vi "校准设置页.vi"() -> ()   [LabVIEW 2016, in "斯坦道氨氮V2.lvlib"]
uses:
  <vilib>/ptbypt/NI_PtbyPt.lvlib
panel:
  in  "校准任务":bool
  in  "历史数据导入":T1(radio)
  out "刷新时间":string
  out "模型刷新":bool
  in  "校准按钮":T1(radio)
  in  "仪器写入":bool
  in  "辅助计算":bool
  in  "曲线模型":T2={"标液浓度1"=0.0, "测量吸光度1"=0.0, "样品1启用"=FALSE, "标液浓度2"=0.0, "测量吸光度2"=0.0, "样品2启用"=FALSE, "标液浓度3"=0.0, "测量吸光度3"=0.0, "样品3启用"=FALSE, "标液浓度4"=0.0, "测量吸光度4"=0.0, "样品4启用"=FALSE, "标液浓度5"=0.0, "测量吸光度5"=0.0, "样品5启用"=FALSE, "模型"=enum."线性", "精度"=4.0, "XY图"=[], "拟合公式"="", "r^2"=0.0, "标样一校准时间"=timestamp(0 s since 1904-01-01), "标样二校准时间"=timestamp(0 s since 1904-01-01), "标样三校准时间"=timestamp(0 s since 1904-01-01), "标样四校准时间"=timestamp(0 s since 1904-01-01), "标样五校准时间"=timestamp(0 s since 1904-01-01), "二次方程"={"c"=0.0, "x"=0.0, "x^2"=0.0}, "标定时间"=timestamp(0 s since 1904-01-01)} {"标定时间" format="%<%y/%m/%d %H:%M:%S>T"; "标样五校准时间" format="%<%y/%m/%d %H:%M:%S>T"; "标样四校准时间" format="%<%y/%m/%d %H:%M:%S>T"; "标样三校准时间" format="%<%y/%m/%d %H:%M:%S>T"; "标样二校准时间" format="%<%y/%m/%d %H:%M:%S>T"; "标样一校准时间" format="%<%y/%m/%d %H:%M:%S>T"; "r^2" format="%.7f"; "测量吸光度5" format="%#.6f"; "测量吸光度4" format="%#.6f"; "测量吸光度3" format="%#.6f"; "测量吸光度2" format="%#.6f"; "测量吸光度1" format="%#.6f"}
  in  "测量模式":enum16{"跨度核查", "水样测量", "零点核查", "标样核查", "加标回收"}(ring)
  in  "参数下拉列表":u16(ring) items=["氨氮"=3, "CODMn"=21]
  in  "量程下拉列表":enum16{"低量程", "高量程"}(ring)
  # "校准时间"
  # "标液浓度"
  # "吸光值"
  # "标样一"
  # "标样二"
  # "标样三"
  # "零点"
  # "跨度"
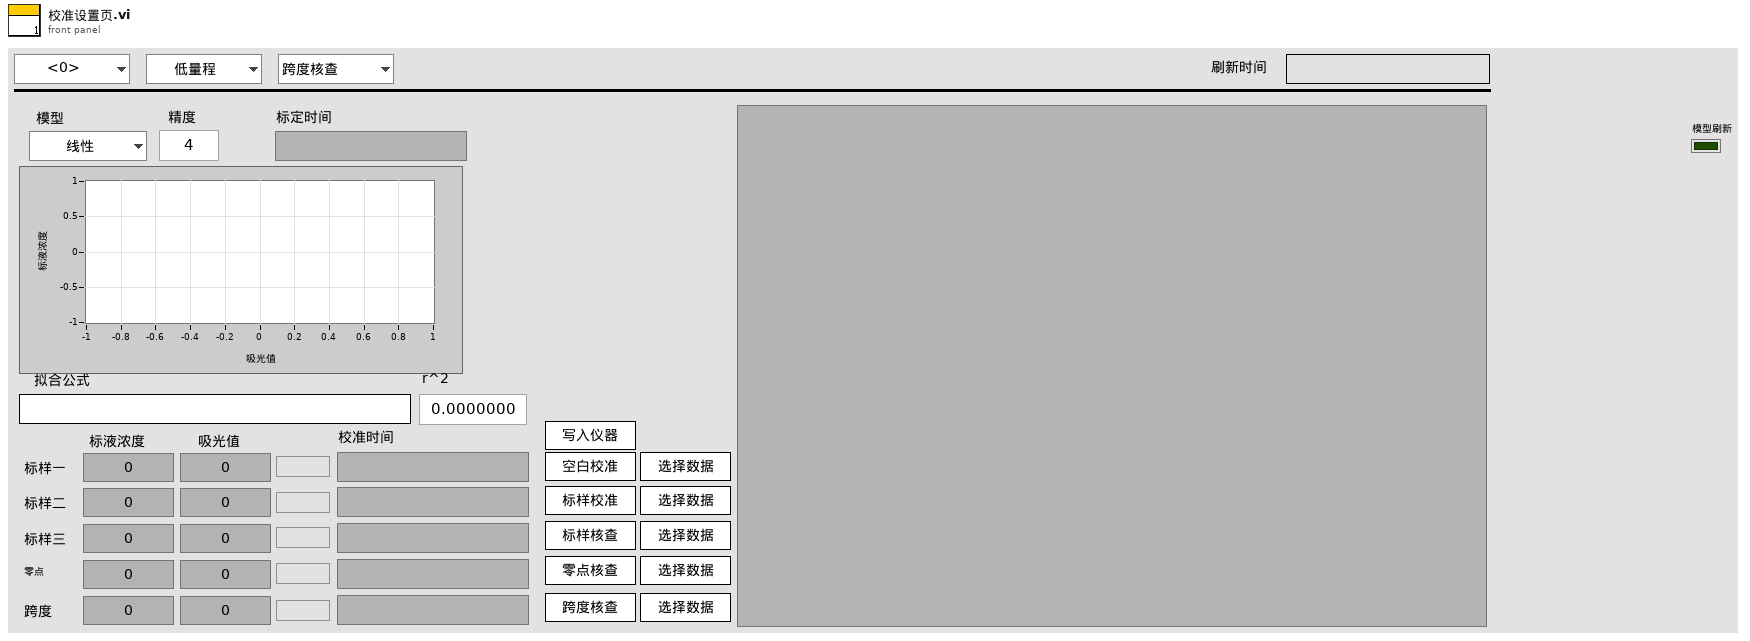
[diagram p1: front panel]
types:
  T1 = enum32{"未选择", "空白校准", "标样校准", "标样核查", "零点核查", "跨度核查"}
  T2 = cluster{"标液浓度1":dbl, "测量吸光度1":dbl, "样品1启用":bool, "标液浓度2":dbl, "测量吸光度2":dbl, "样品2启用":bool, "标液浓度3":dbl, "测量吸光度3":dbl, "样品3启用":bool, "标液浓度4":dbl, "测量吸光度4":dbl, "样品4启用":bool, "标液浓度5":dbl, "测量吸光度5":dbl, "样品5启用":bool, "模型":enum32{"线性", "多项式"}, "精度":dbl, "XY图":cluster{"X Values":dbl[], "Y Values":dbl[]}[], "拟合公式":string, "r^2":dbl, "标样一校准时间":timestamp, "标样二校准时间":timestamp, "标样三校准时间":timestamp, "标样四校准时间":timestamp, "标样五校准时间":timestamp, "二次方程":cluster{"c":dbl, "x":dbl, "x^2":dbl}, "标定时间":timestamp}
  T3 = typedef "斯坦道氨氮V2.lvlib/校准任务.ctl" = cluster{"id":u16, "任务类型":enum16{"未选择", "空白校准", "标样校准", "标样核查", "零点核查", "跨度核查"}, "量程下拉列表":enum16{"低量程", "高量程"}, "状态":enum16{"已执行", "待执行", "执行中", "停止"}, "标液浓度":dbl, "吸光值":dbl, "校准时间":timestamp}
  T4 = enum8{"Enabled", "Disabled", "Disabled and Grayed Out"}
  T5 = enum16{"跨度核查", "水样测量", "零点核查", "标样核查", "加标回收", "快捷测试", "空白校准", "标样校准"}
  T6 = typedef "LVStringsAndValuesArrayTypeDef_U16.ctl" = cluster{"String":string, "Value":u16}[]
  T7 = cluster{"标液浓度1":dbl, "测量吸光度1":dbl, "样品1启用":bool, "标液浓度2":dbl, "测量吸光度2":dbl, "样品2启用":bool, "标液浓度3":dbl, "测量吸光度3":dbl, "样品3启用":bool, "标液浓度4":dbl, "测量吸光度4":dbl, "样品4启用":bool, "标液浓度5":dbl, "测量吸光度5":dbl, "样品5启用":bool, "模型":enum32{"线性", "多项式"}, "精度":dbl, "XY图":cluster{"X Values":dbl[], "Y Values":dbl[]}[], "拟合公式":string, "r^2":dbl, "标样一校准时间":timestamp, "标样二校准时间":timestamp, "标样三校准时间":timestamp, "标样四校准时间":timestamp, "标样五校准时间":timestamp, "二次方程":cluster{"c":dbl, "x":dbl, "x^2":dbl}, "标定时间":timestamp}[]
  T8 = cluster{"时间":timestamp, "标液值":dbl, "检测值":dbl, "吸光值":dbl}
  T9 = enum32{"Bad", "Idle", "Run top level", "Running"}
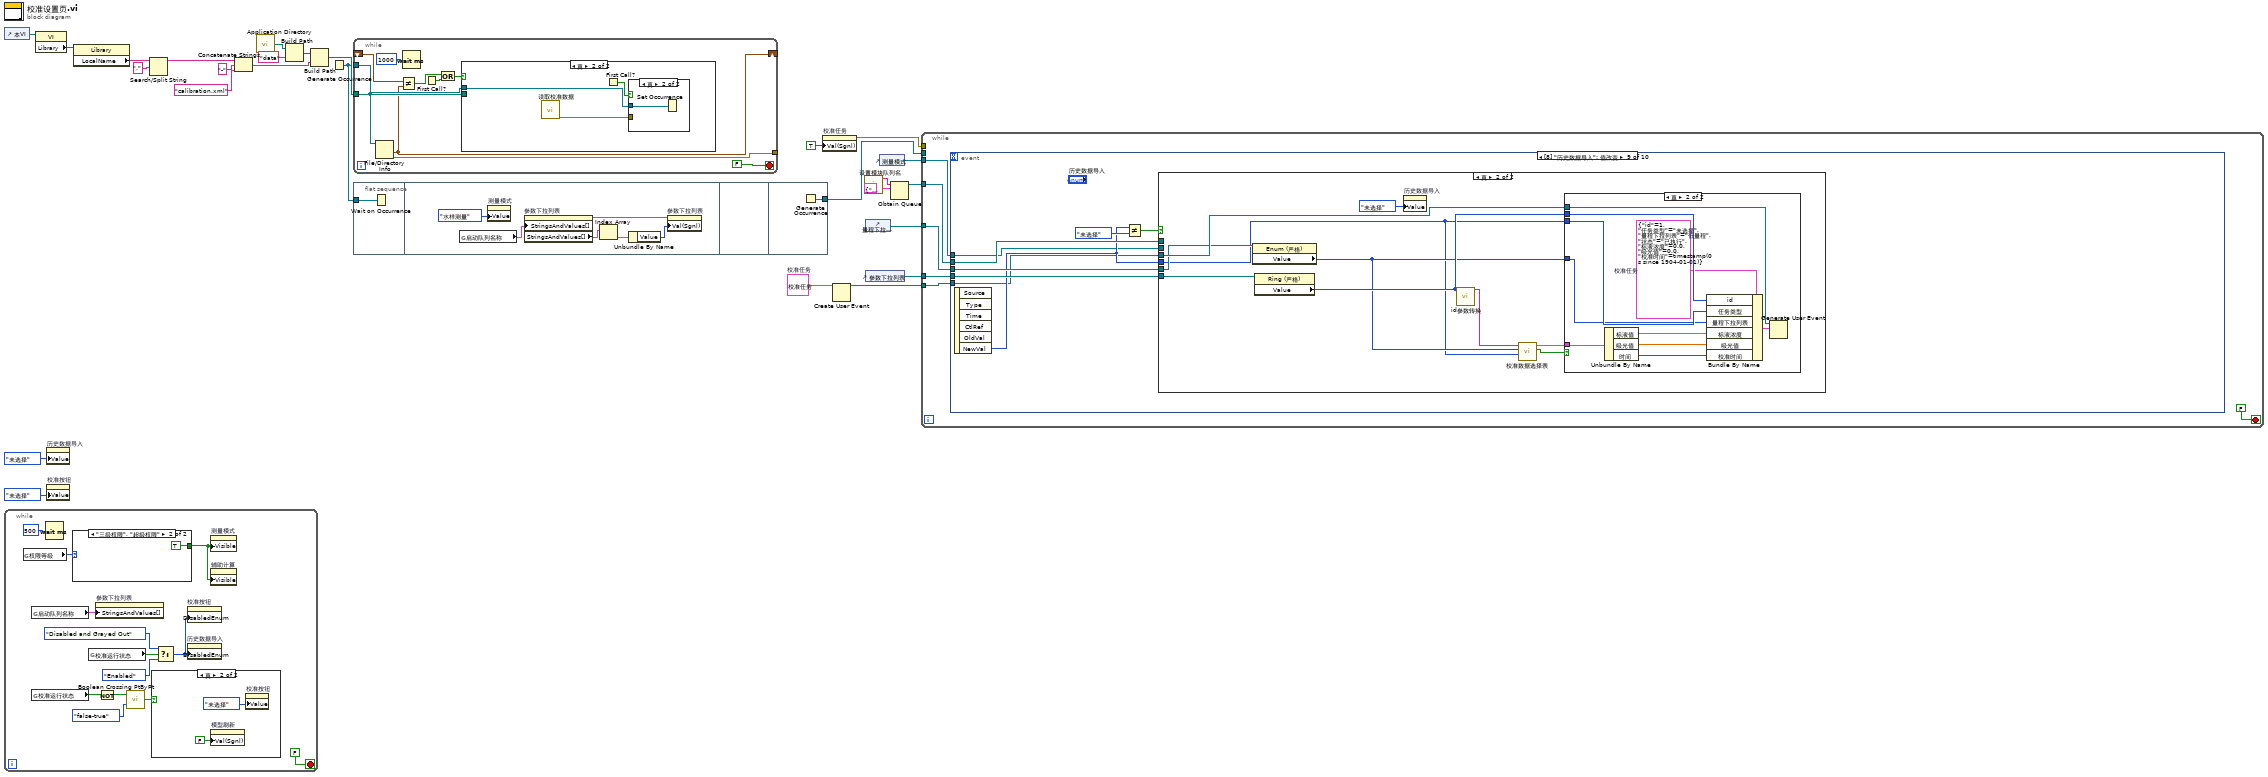
[diagram p0: block diagram]
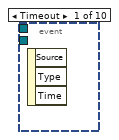
[diagram p4: hidden frame]
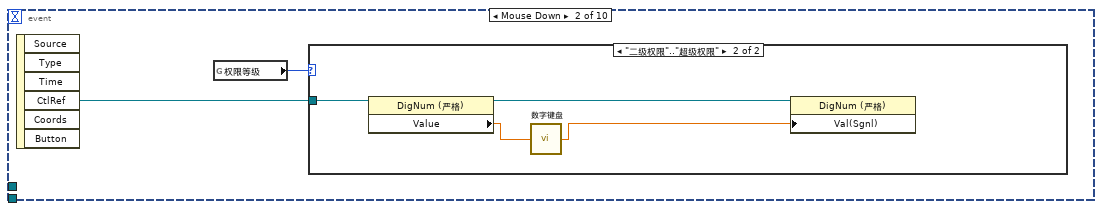
[diagram p5: hidden frame]
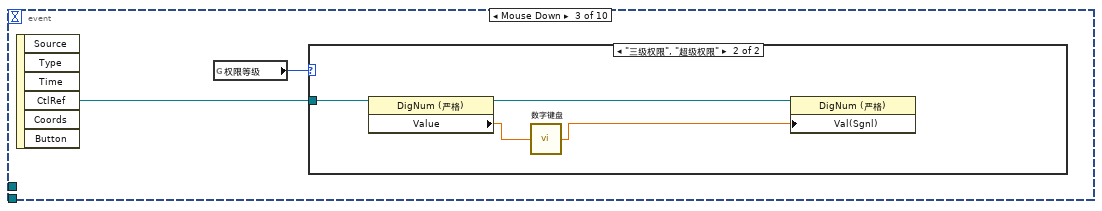
[diagram p7: hidden frame]
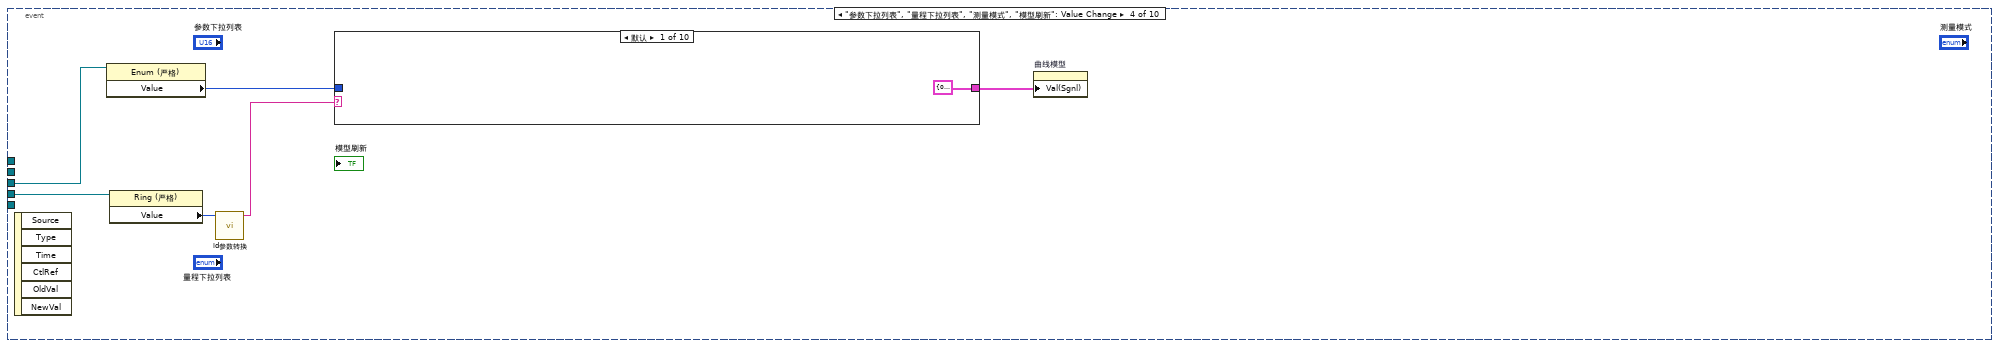
[diagram p9: hidden frame]
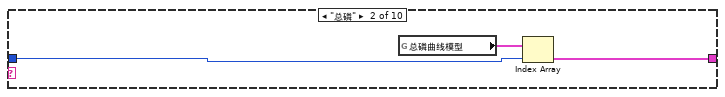
[diagram p10: hidden frame]
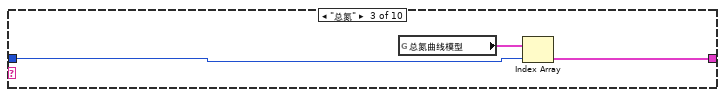
[diagram p11: hidden frame]
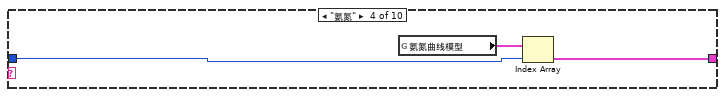
[diagram p12: hidden frame]
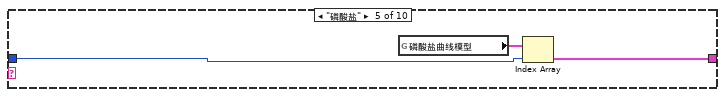
[diagram p13: hidden frame]
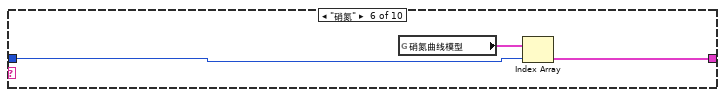
[diagram p14: hidden frame]
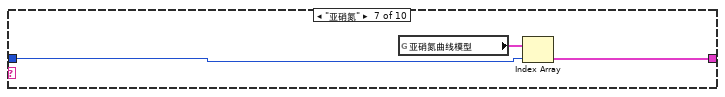
[diagram p15: hidden frame]
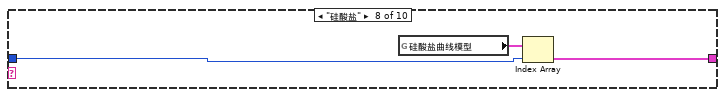
[diagram p16: hidden frame]
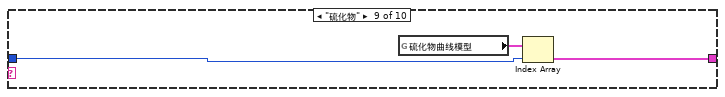
[diagram p17: hidden frame]
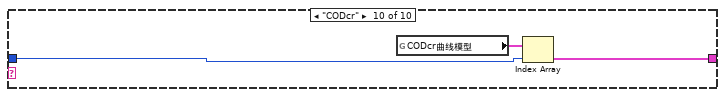
[diagram p18: hidden frame]
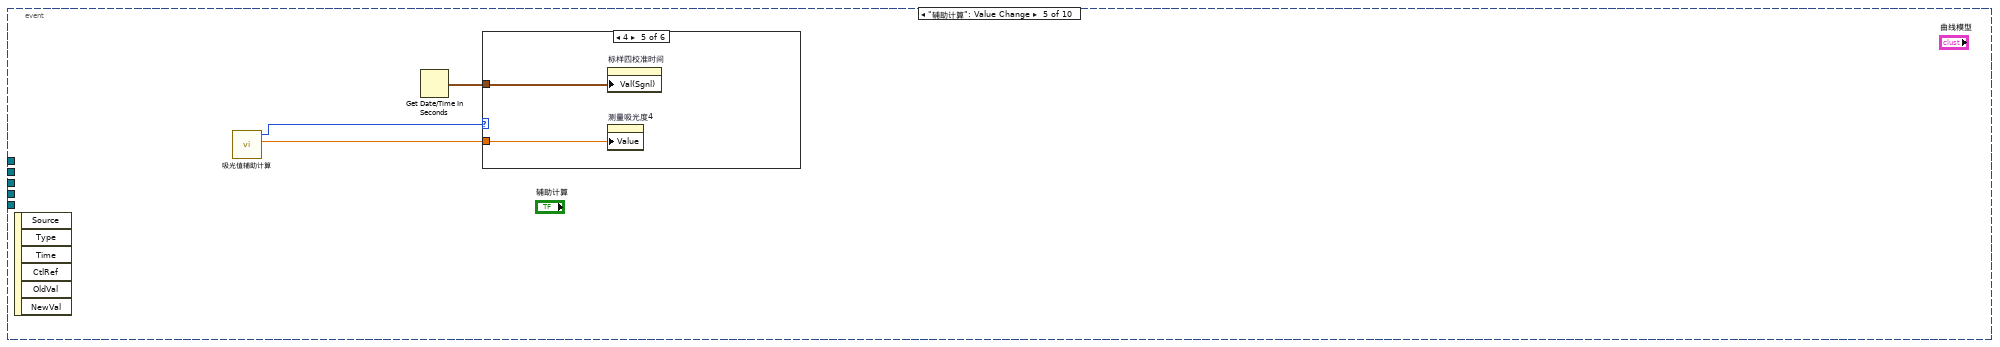
[diagram p19: hidden frame]
diagram:
  w3 = T3 {"id"=1, "任务类型"=enum."未选择", "量程下拉列表"=enum."低量程", "状态"=enum."已执行", "标液浓度"=0.0, "吸光值"=0.0, "校准时间"=timestamp(0 s since 1904-01-01)}  # 校准任务
  n1 = control-ref of="本VI"() -> (w14:refnum<vi>)
  n2 = while {
    stop <- FALSE stop-if-true
    n3 = global read "VAR总磷总氮全局变量.vi" "权限等级"() -> (w37:enum16{"一级权限", "二级权限", "三级权限", "超级权限"})
    n4 = global read "总磷总氮断电保存全局变量.vi" "启动队列名称"() -> (w34:cluster{"String":string, "Value":u16}[])
    n5 = global read "VAR总磷总氮全局变量.vi" "校准运行状态"() -> (w33:bool)
    n6 = Wait (ms)(milliseconds to wait=u32 500 ("等待时间（毫秒）")) -> ()  [unwired: 1 out]
    n7 = case shown="\"三级权限\", \"超级权限\"" w37 {
      tunnel: [_ TRUE ("可见")] -> w27
      frame "一级权限", Default {
        n8 = property on="测量模式" class="Enum (严格)"("Value"=T5."水样测量" ("测量模式")) -> ()  [unwired: 2 in, 2 out]
      }
      frame "三级权限", "超级权限" {
      }
    }
    n9 = global read "VAR总磷总氮全局变量.vi" "校准运行状态"() -> (w31:bool)
    n10 = property on="参数下拉列表" class="Ring (严格)"("StringsAndValues[]"=w34) -> ()  [unwired: 2 in, 2 out]
    n11 = Not(x=w33) -> (.not. x?=w32:bool)
    n12 = call <vilib>:"Boolean Crossing PtByPt.vi"("direction"=enum16{"either", "false-true", "true-false"}."false-true", "input"=w32) -> ("crossing"=w35:bool)  [unwired: 1 in]
    n13 = case shown="真" w35 {
      frame False {
      }
      frame True {
        n14 = property on="模型刷新" class="Bool (严格)"("Val(Sgnl)"=FALSE ("值(信号)")) -> ()  [unwired: 2 in, 2 out]
        n15 = property on="校准按钮" class="RadioBtnsControl (严格)"("Value"=T1."未选择" ("校准按钮")) -> ()  [unwired: 2 in, 2 out]
      }
    }
    n16 = Select(t=T4."Disabled and Grayed Out" ("禁用"), s=w31, f=T4."Enabled" ("禁用")) -> (s? t:f=w29:T4)
    n17 = property on="校准按钮" class="RadioBtnsControl (严格)"("DisabledEnum"=w29) -> ()  [unwired: 2 in, 2 out]
    n18 = property on="历史数据导入" class="RadioBtnsControl (严格)"("DisabledEnum"=w29) -> ()  [unwired: 2 in, 2 out]
    n19 = property on="测量模式" class="Enum (严格)"("Visible"=w27) -> ()  [unwired: 2 in, 2 out]
    n20 = property on="辅助计算" class="Bool"("Visible"=w27) -> ()  [unwired: 2 in, 2 out]
  }
  n21 = property class="VI"(reference=w14) -> ("Library"=w15:refnum<vi>)  [unwired: 1 in, 2 out]
  n22 = property on="历史数据导入" class="RadioBtnsControl (严格)"("Value"=T1."未选择" ("历史数据导入")) -> ()  [unwired: 2 in, 2 out]
  n23 = property on="校准按钮" class="RadioBtnsControl (严格)"("Value"=T1."未选择" ("校准按钮")) -> ()  [unwired: 2 in, 2 out]
  n24 = property class="Library"(reference=w15) -> ("LocalName"=w12:string)  [unwired: 1 in, 2 out]
  n25 = Search/Split String(string=w12, search string/char (-)="." ("搜索字符串/字符(-)")) -> (substring before match=w10:string)  [unwired: 1 in, 2 out]
  n26 = Concatenate Strings(w10, "-" ("字符串"), "calibration.xml" ("名称或相对路径")) -> (w7:string)
  n27 = call <vilib>:"Application Directory.vi"() -> ("Application Directory"=w16:path)
  n28 = Build Path(base path=w16, name or relative path="data" ("名称或相对路径")) -> (appended path=w13:path)
  n29 = Build Path(base path=w13, name or relative path=w7) -> (appended path=w6:path)
  n30 = Generate Occurrence() -> (w5:refnum<k4>)
  n31 = while {
    shift-right: [w44] -> _
    shift-left: _ -> [w52]
    tunnel: w6 -> [w50]
    tunnel: [w48] -> _
    tunnel: w5 -> [w47]
    stop <- FALSE stop-if-true
    n32 = File/Directory Info(path=w50) -> (last mod=w44:timestamp, error out=w48:errorcluster)  [unwired: 1 in, 5 out]
    n33 = Not Equal?(x=w52, y=w44) -> (x != y?=w51:bool)
    n34 = Wait (ms)(milliseconds to wait=u32 1000 ("等待时间（毫秒）")) -> ()  [unwired: 1 out]
    n35 = First Call?() -> (First Call?: T/F=w45:bool)
    n36 = Or(x=w51, y=w45) -> (x .or. y?=w46:bool)
    n37 = case shown="真" w46 {
      tunnel: w50 -> [_ _]
      tunnel: w47 -> [_ w56]
      frame False {
      }
      frame True {
        n38 = call "读取校准数据.vi"() -> ("错误输出"=w55:errorcluster)  [unwired: 11 in]
        n39 = First Call?() -> (First Call?: T/F=w54:bool)
        n40 = case shown="真" w54 {
          tunnel: w56 -> [_ w57]
          tunnel: w55 -> [_ _]
          frame False {
          }
          frame True {
            n41 = Set Occurrence(w57) -> ()
          }
        }
      }
    }
  }
  n42 = flat-sequence {
    tunnel: w5 -> [w58]
    tunnel: [w65] -> w26
    frame #0 {
      n43 = Wait on Occurrence(2:w58) -> ()  [unwired: 2 in, 1 out]
    }
    frame #1 {
      n44 = global read "总磷总氮断电保存全局变量.vi" "启动队列名称"() -> (w60:cluster{"String":string, "Value":u16}[])
      n45 = property on="测量模式" class="Enum (严格)"("Value"=T5."水样测量" ("测量模式")) -> ()  [unwired: 2 in, 2 out]
      n46 = property on="参数下拉列表" class="Ring (严格)"("StringsAndValues[]"=w60) -> (error out=w63:errorcluster, "StringsAndValues[]"=w61:T6)  [unwired: 2 in, 1 out]
      n47 = Index Array(array=w61) -> (element=w62:cluster{"String":string, "Value":u16})  [unwired: 1 in]
      n48 = Unbundle By Name(w62) -> ("Value"=w64:u16)
      n49 = property on="参数下拉列表" class="Ring (严格)"(error in=w63, "Val(Sgnl)"=w64) -> ()  [unwired: 1 in, 2 out]
    }
    frame #2 {
    }
    frame #3 {
      n50 = Generate Occurrence() -> (w65:refnum<k4>)
    }
  }
  n51 = property on="校准任务" class="Bool (严格)"("Val(Sgnl)"=TRUE ("值(信号)")) -> (error out=w2:errorcluster)  [unwired: 2 in, 1 out]
  n52 = Create User Event(user event datatype=w3) -> (user event=w4:refnum<user-event>)  [unwired: 1 in, 1 out]
  n53 = call "设置模块队列名.vi"() -> ("Msg"=w24:string)  [unwired: 5 in]
  n54 = control-ref of="量程下拉列表"() -> (w19:refnum<vi>)
  n55 = control-ref of="参数下拉列表"() -> (w21:refnum<vi>)
  n56 = control-ref of="测量模式"() -> (w20:refnum<vi>)
  n57 = Obtain Queue(name (unnamed)=w24, element data type=cluster{"命令":string, "data":variant} {"命令"="", "data"=variant}) -> (queue out=w23:refnum<queue>)  [unwired: 3 in, 2 out]
  n58 = while {
    tunnel: w26 -> [_]
    tunnel: w21 -> [w70]
    tunnel: w20 -> [w69]
    tunnel: w19 -> [w68]
    tunnel: w23 -> [w67]
    tunnel: w4 -> [w66]
    tunnel: w2 -> [_]
    stop <- FALSE stop-if-true
    n59 = event shown="[8] \"历史数据导入\": 值改变" {
      selector: _ -> [_ _ _ _ _ _ _ _ _ _]
      dyn-events: _ -> [_ _ _ _ _ _ _ _ _ _]
      timeout: _ -> [_ _ _ _ _ _ _ _ _ _]
      tunnel: w70 -> [_ _ _ w88 _ w143 w188 w242 w270 _]
      tunnel: w69 -> [_ _ _ _ _ w141 _ w237 w265 _]
      tunnel: w68 -> [_ _ _ w86 _ w139 w186 w241 w269 _]
      tunnel: w67 -> [_ _ _ _ _ _ _ w243 w271 _]
      tunnel: w66 -> [_ _ _ _ _ _ _ w236 w264 w293]
      event Timeout {
        n60 = event-data() -> ()  [unwired: 1 in, 3 out]
      }
      event "曲线模型.标液浓度1", "曲线模型.标液浓度2", "曲线模型.标液浓度3", "曲线模型.标液浓度4", "曲线模型.标液浓度5", "曲线模型.精度": Mouse Down {
        n61 = event-data() -> ("CtlRef"=w73:refnum<vi>)  [unwired: 1 in, 5 out]
        n62 = global read "VAR总磷总氮全局变量.vi" "权限等级"() -> (w72:enum16{"一级权限", "二级权限", "三级权限", "超级权限"})
        n63 = case shown="\"二级权限\"..\"超级权限\"" w72 {
          tunnel: w73 -> [_ w77]
          frame "一级权限", Default {
          }
          frame "二级权限".."超级权限" {
            n64 = property class="DigNum (严格)"(reference=w77) -> (reference out=w75:refnum<vi>, "Value"=w76:dbl)  [unwired: 1 in, 1 out]
            n65 = call "数字键盘.vi"("OldNumber"=w76) -> ("NewNumber"=w74:dbl)
            n66 = property class="DigNum (严格)"(reference=w75, "Val(Sgnl)"=w74) -> ()  [unwired: 1 in, 2 out]
          }
        }
      }
      event "曲线模型.测量吸光度1", "曲线模型.测量吸光度2", "曲线模型.测量吸光度3", "曲线模型.测量吸光度4", "曲线模型.测量吸光度5": Mouse Down {
        n67 = event-data() -> ("CtlRef"=w79:refnum<vi>)  [unwired: 1 in, 5 out]
        n68 = global read "VAR总磷总氮全局变量.vi" "权限等级"() -> (w78:enum16{"一级权限", "二级权限", "三级权限", "超级权限"})
        n69 = case shown="\"三级权限\", \"超级权限\"" w78 {
          tunnel: w79 -> [_ w83]
          frame "一级权限", Default {
          }
          frame "三级权限", "超级权限" {
            n70 = property class="DigNum (严格)"(reference=w83) -> (reference out=w81:refnum<vi>, "Value"=w82:dbl)  [unwired: 1 in, 1 out]
            n71 = call "数字键盘.vi"("OldNumber"=w82) -> ("NewNumber"=w80:dbl)
            n72 = property class="DigNum (严格)"(reference=w81, "Val(Sgnl)"=w80) -> ()  [unwired: 1 in, 2 out]
          }
        }
      }
      event "参数下拉列表", "量程下拉列表", "测量模式", "模型刷新": Value Change {
        n73 = event-data() -> ()  [unwired: 1 in, 6 out]
        n74 = property class="Enum (严格)"(reference=w86) -> ("Value"=w84:enum16{"低量程", "高量程"})  [unwired: 1 in, 2 out]
        n75 = property class="Ring (严格)"(reference=w88) -> ("Value"=w89:u16)  [unwired: 1 in, 2 out]
        n76 = call "id参数转换.vi"("id"=w89) -> ("table输出"=w87:string)  [unwired: 9 in, 1 out]
        n77 = case shown="默认" w87 {
          tunnel: w84 -> [_ w91 w94 w97 w100 w103 w106 w109 w112 w115]
          tunnel: [T2 {"标液浓度1"=0.0, "测量吸光度1"=0.0, "样品1启用"=FALSE, "标液浓度2"=0.0, "测量吸光度2"=0.0, "样品2启用"=FALSE, "标液浓度3"=0.0, "测量吸光度3"=0.0, "样品3启用"=FALSE, "标液浓度4"=0.0, "测量吸光度4"=0.0, "样品4启用"=FALSE, "标液浓度5"=0.0, "测量吸光度5"=0.0, "样品5启用"=FALSE, "模型"=enum."线性", "精度"=0.0, "XY图"=[], "拟合公式"="", "r^2"=0.0, "标样一校准时间"=timestamp(0 s since 1904-01-01), "标样二校准时间"=timestamp(0 s since 1904-01-01), "标样三校准时间"=timestamp(0 s since 1904-01-01), "标样四校准时间"=timestamp(0 s since 1904-01-01), "标样五校准时间"=timestamp(0 s since 1904-01-01), "二次方程"={"c"=0.0, "x"=0.0, "x^2"=0.0}, "标定时间"=timestamp(0 s since 1904-01-01)} ("总磷曲线模型") w92 w95 w98 w101 w104 w107 w110 w113 w116] -> w85
          frame Default {
          }
          frame "总磷" {
            n78 = global read "校准数据全局变量.vi" "总磷曲线模型"() -> (w93:T7)
            n79 = Index Array(array=w93, index=w91) -> (element=w92:T2)
          }
          frame "总氮" {
            n80 = global read "校准数据全局变量.vi" "总氮曲线模型"() -> (w96:T7)
            n81 = Index Array(array=w96, index=w94) -> (element=w95:T2)
          }
          frame "氨氮" {
            n82 = global read "校准数据全局变量.vi" "氨氮曲线模型"() -> (w99:T7)
            n83 = Index Array(array=w99, index=w97) -> (element=w98:T2)
          }
          frame "磷酸盐" {
            n84 = global read "校准数据全局变量.vi" "磷酸盐曲线模型"() -> (w102:T7)
            n85 = Index Array(array=w102, index=w100) -> (element=w101:T2)
          }
          frame "硝氮" {
            n86 = global read "校准数据全局变量.vi" "硝氮曲线模型"() -> (w105:T7)
            n87 = Index Array(array=w105, index=w103) -> (element=w104:T2)
          }
          frame "亚硝氮" {
            n88 = global read "校准数据全局变量.vi" "亚硝氮曲线模型"() -> (w108:T7)
            n89 = Index Array(array=w108, index=w106) -> (element=w107:T2)
          }
          frame "硅酸盐" {
            n90 = global read "校准数据全局变量.vi" "硅酸盐曲线模型"() -> (w111:T7)
            n91 = Index Array(array=w111, index=w109) -> (element=w110:T2)
          }
          frame "硫化物" {
            n92 = global read "校准数据全局变量.vi" "硫化物曲线模型"() -> (w114:T7)
            n93 = Index Array(array=w114, index=w112) -> (element=w113:T2)
          }
          frame "CODcr" {
            n94 = global read "校准数据全局变量.vi" "CODcr曲线模型"() -> (w117:T7)
            n95 = Index Array(array=w117, index=w115) -> (element=w116:T2)
          }
        }
        n96 = property on="曲线模型" class="Clust (严格)"("Val(Sgnl)"=w85) -> ()  [unwired: 2 in, 2 out]
      }
      event "辅助计算": Value Change {
        n97 = event-data() -> ()  [unwired: 1 in, 6 out]
        n98 = call "吸光值辅助计算.vi"() -> ("X"=w119:dbl, "吸光值导出"=w120:u16)  [unwired: 10 in]
        n99 = Get Date/Time In Seconds() -> (seconds since 1Jan1904=w118:timestamp)
        n100 = case shown="4" w120 {
          tunnel: w119 -> [_ w122 w124 w126 w128 w130]
          tunnel: w118 -> [_ w121 w123 w125 w127 w129]
          frame 0, Default {
          }
          frame 1 {
            n101 = property on="标样一校准时间" class="AbsTime (严格)"("Val(Sgnl)"=w121) -> ()  [unwired: 2 in, 2 out]
            n102 = property on="测量吸光度1" class="DigNum (严格)"("Value"=w122) -> ()  [unwired: 2 in, 2 out]
          }
          frame 2 {
            n103 = property on="标样二校准时间" class="AbsTime (严格)"("Val(Sgnl)"=w123) -> ()  [unwired: 2 in, 2 out]
            n104 = property on="测量吸光度2" class="DigNum (严格)"("Value"=w124) -> ()  [unwired: 2 in, 2 out]
          }
          frame 3 {
            n105 = property on="标样三校准时间" class="AbsTime (严格)"("Val(Sgnl)"=w125) -> ()  [unwired: 2 in, 2 out]
            n106 = property on="测量吸光度3" class="DigNum (严格)"("Value"=w126) -> ()  [unwired: 2 in, 2 out]
          }
          frame 4 {
            n107 = property on="标样四校准时间" class="AbsTime (严格)"("Val(Sgnl)"=w127) -> ()  [unwired: 2 in, 2 out]
            n108 = property on="测量吸光度4" class="DigNum (严格)"("Value"=w128) -> ()  [unwired: 2 in, 2 out]
          }
          frame 5 {
            n109 = property on="标样五校准时间" class="AbsTime (严格)"("Val(Sgnl)"=w129) -> ()  [unwired: 2 in, 2 out]
            n110 = property on="测量吸光度5" class="DigNum (严格)"("Value"=w130) -> ()  [unwired: 2 in, 2 out]
          }
        }
      }
      event "仪器写入": Value Change {
        n111 = event-data() -> ()  [unwired: 1 in, 6 out]
        n112 = property class="Enum (严格)"(reference=w141) -> ("Value"=w140:enum16{"跨度核查", "水样测量", "零点核查", "标样核查", "加标回收"})  [unwired: 1 in, 2 out]
        n113 = property class="Enum (严格)"(reference=w139) -> ("Value"=w138:enum16{"低量程", "高量程"})  [unwired: 1 in, 2 out]
        n114 = property class="Ring (严格)"(reference=w143) -> ("Value"=w142:u16)  [unwired: 1 in, 2 out]
        n115 = property on="二次方程" class="Clust (严格)"() -> ("Value"=w132:cluster{"c":dbl, "x":dbl, "x^2":dbl})  [unwired: 2 in, 2 out]
        n116 = Unbundle By Name(w132) -> ("x^2"=w134:dbl, "x"=w135:dbl, "c"=w136:dbl)
        n117 = Bundle By Name(cluster=cluster{"X^2":dbl, "X":dbl, "b":dbl} {"X^2"=0.0, "X"=0.0, "b"=0.0} ("公式"), "X^2"=w134, "X"=w135, "b"=w136) -> (w131:cluster{"X^2":dbl, "X":dbl, "b":dbl})
        n118 = global read "VAR总磷总氮全局变量.vi" "权限等级"() -> (w137:enum16{"一级权限", "二级权限", "三级权限", "超级权限"})
        n119 = case shown="\"一级权限\", 默认" w137 {
          tunnel: w142 -> [w152 w184]
          tunnel: w140 -> [w151 w183]
          tunnel: w138 -> [w150 w182]
          tunnel: w131 -> [w144 w181]
          frame "一级权限", Default {
            n120 = Cluster To Array(cluster=w144) -> (array=w149:dbl[])
            n121 = Add Array Elements(numeric array=w149) -> (sum=w148:dbl)
            n122 = Equal To 0?(x=w148) -> (x = 0?=w146:bool)
            n123 = Not A Number/Path/Refnum?(number/path/refnum=w148) -> (NaN/Path/Refnum?=w147:bool)
            n124 = Or(x=w146, y=w147) -> (x .or. y?=w145:bool)
            n125 = case shown="假" w145 {
              tunnel: w152 -> [w158 _]
              tunnel: w151 -> [w157 _]
              tunnel: w150 -> [w156 _]
              tunnel: w144 -> [w153 _]
              frame False {
                n126 = Two Button Dialog(message="请再一次确认是否导入" ("消息")) -> (T button?=w154:bool)  [unwired: 2 in]
                n127 = case shown="真" w154 {
                  tunnel: w158 -> [_ w160]
                  tunnel: w157 -> [_ w166]
                  tunnel: w156 -> [_ w159]
                  tunnel: w153 -> [_ w161]
                  frame False {
                  }
                  frame True {
                    n128 = for {
                      N: 8 -> [_]
                      tunnel: w160 -> [w172]
                      tunnel: w166 -> [_]
                      tunnel: w159 -> [w171]
                      shift-right: [w170] -> w164
                      shift-left: errorcluster {"status"=FALSE, "code"=0, "source"=""} ("error out") -> [w167]
                      tunnel: w161 -> [w168]
                      i -> [w169]
                      n129 = call "公式写入.vi"("公式"=w168, "error in (no error)"=w167, "量程下拉列表"=w171, "测量模式"=w169, "参数下拉列表"=w172) -> ("error out"=w170:errorcluster)  [unwired: 6 in]
                    }
                    n130 = case shown="无错误" w164 {
                      tunnel: ["写入成功" "写入失败"] -> w165
                      tunnel: w160 -> [w176 _]
                      tunnel: w159 -> [w175 _]
                      frame No Error {
                        n131 = Get Date/Time In Seconds() -> (seconds since 1Jan1904=w177:timestamp)
                        n132 = property on="标定时间" class="AbsTime (严格)"("Val(Sgnl)"=w177) -> (error out=w173:errorcluster)  [unwired: 2 in, 1 out]
                        n133 = property on="曲线模型" class="Clust (严格)"(error in=w173) -> ("Value"=w174:T2)  [unwired: 1 in, 2 out]
                        n134 = call "校准记录.vi"("曲线模型"=w174, "量程"=w175, "校准参数"=w176) -> ()  [unwired: 8 in, 1 out]
                      }
                      frame Error {
                      }
                    }
                    n135 = One Button Dialog(message=w165) -> ()  [unwired: 1 in, 1 out]
                  }
                }
              }
              frame True {
                n136 = One Button Dialog(message="校准数据异常，请重新校准！" ("消息")) -> ()  [unwired: 1 in, 1 out]
              }
            }
          }
          frame "三级权限", "超级权限" {
            n137 = call "公式复合写入.vi"("公式"=w181, "量程下拉列表"=w182, "测量模式"=w183, "参数下拉列表"=w184) -> ()  [unwired: 8 in]
          }
        }
      }
      event "曲线模型": Value Change {
        n138 = event-data() -> ()  [unwired: 1 in, 6 out]
        n139 = flat-sequence {
          tunnel: [w193] -> w189
          tunnel: w188 -> [w193]
          tunnel: [w192] -> w187
          tunnel: w186 -> [w192]
          tunnel: w189 -> [w199]
          tunnel: w187 -> [w196]
          frame #0 {
            n140 = property on="曲线模型" class="Clust (严格)"() -> ("Value"=w191:T2)  [unwired: 2 in, 2 out]
            n141 = call "曲线模型计算.vi"("曲线模型"=w191) -> ("输出簇"=w190:T2)  [unwired: 10 in]
            n142 = property on="曲线模型" class="Clust (严格)"("Value"=w190) -> ()  [unwired: 2 in, 2 out]
          }
          frame #1 {
            n143 = property class="Enum (严格)"(reference=w196) -> ("Value"=w195:enum16{"低量程", "高量程"})  [unwired: 1 in, 2 out]
            n144 = property class="Ring (严格)"(reference=w199) -> ("Value"=w198:u16)  [unwired: 1 in, 2 out]
            n145 = call "id参数转换.vi"("id"=w198) -> ("table输出"=w197:string)  [unwired: 9 in, 1 out]
            n146 = property on="曲线模型" class="Clust (严格)"() -> ("Value"=w194:T2)  [unwired: 2 in, 2 out]
            n147 = case shown="\"总磷\"" w197 {
              tunnel: w194 -> [_ w201 w207 w210 w213 w217 w221 w225 w229 w234]
              tunnel: w195 -> [_ w200 w204 w208 w212 w216 w220 w224 w228 w232]
              frame Default {
              }
              frame "总磷" {
                n148 = global read "校准数据全局变量.vi" "总磷曲线模型"() -> (w202:T7)
                n149 = Replace Array Subset(array=w202, new element=w201, index=w200) -> (w203:T7)
                n150 = global write "校准数据全局变量.vi" "总磷曲线模型"(w203) -> ()
              }
              frame "总氮" {
                n151 = global read "校准数据全局变量.vi" "总氮曲线模型"() -> (w206:T7)
                n152 = Replace Array Subset(array=w206, new element=w207, index=w204) -> (w205:T7)
                n153 = global write "校准数据全局变量.vi" "总氮曲线模型"(w205) -> ()
              }
              frame "氨氮" {
                n154 = global read "校准数据全局变量.vi" "氨氮曲线模型"() -> (w211:T7)
                n155 = Replace Array Subset(array=w211, new element=w210, index=w208) -> (w209:T7)
                n156 = global write "校准数据全局变量.vi" "氨氮曲线模型"(w209) -> ()
              }
              frame "磷酸盐" {
                n157 = global read "校准数据全局变量.vi" "磷酸盐曲线模型"() -> (w215:T7)
                n158 = Replace Array Subset(array=w215, new element=w213, index=w212) -> (w214:T7)
                n159 = global write "校准数据全局变量.vi" "磷酸盐曲线模型"(w214) -> ()
              }
              frame "硝氮" {
                n160 = global read "校准数据全局变量.vi" "硝氮曲线模型"() -> (w219:T7)
                n161 = Replace Array Subset(array=w219, new element=w217, index=w216) -> (w218:T7)
                n162 = global write "校准数据全局变量.vi" "硝氮曲线模型"(w218) -> ()
              }
              frame "亚硝氮" {
                n163 = global read "校准数据全局变量.vi" "亚硝氮曲线模型"() -> (w223:T7)
                n164 = Replace Array Subset(array=w223, new element=w221, index=w220) -> (w222:T7)
                n165 = global write "校准数据全局变量.vi" "亚硝氮曲线模型"(w222) -> ()
              }
              frame "硅酸盐" {
                n166 = global read "校准数据全局变量.vi" "硅酸盐曲线模型"() -> (w227:T7)
                n167 = Replace Array Subset(array=w227, new element=w225, index=w224) -> (w226:T7)
                n168 = global write "校准数据全局变量.vi" "硅酸盐曲线模型"(w226) -> ()
              }
              frame "硫化物" {
                n169 = global read "校准数据全局变量.vi" "硫化物曲线模型"() -> (w231:T7)
                n170 = Replace Array Subset(array=w231, new element=w229, index=w228) -> (w230:T7)
                n171 = global write "校准数据全局变量.vi" "硫化物曲线模型"(w230) -> ()
              }
              frame "CODcr" {
                n172 = global read "校准数据全局变量.vi" "CODcr曲线模型"() -> (w235:T7)
                n173 = Replace Array Subset(array=w235, new element=w234, index=w232) -> (w233:T7)
                n174 = global write "校准数据全局变量.vi" "CODcr曲线模型"(w233) -> ()
              }
            }
          }
          frame #2 {
            n175 = call "校准数据写入配置文件.vi"() -> ()  [unwired: 11 in, 1 out]
          }
        }
        n176 = Format Date/Time String() -> (date/time string=→"刷新时间":string)  [unwired: 3 in]
      }
      event "校准按钮": Value Change {
        n177 = event-data() -> ("NewVal"=w238:T1)  [unwired: 1 in, 5 out]
        n178 = Not Equal?(x=w238, y=T1."未选择") -> (x != y?=w239:bool)
        n179 = case shown="真" w239 {
          tunnel: w243 -> [_ _]
          tunnel: w242 -> [_ w253]
          tunnel: w241 -> [_ w252]
          tunnel: w238 -> [_ w248]
          tunnel: w237 -> [_ _]
          tunnel: w236 -> [_ w251]
          frame False {
          }
          frame True {
            w245 = T3 {"id"=1, "任务类型"=enum."未选择", "量程下拉列表"=enum."低量程", "状态"=enum."待执行", "标液浓度"=0.0, "吸光值"=0.0, "校准时间"=timestamp(0 s since 1904-01-01)}  # 校准任务
            n180 = property class="Enum (严格)"(reference=w252) -> ("Value"=w249:enum16{"低量程", "高量程"})  [unwired: 1 in, 2 out]
            n181 = property class="Ring (严格)"(reference=w253) -> ("Value"=w250:u16)  [unwired: 1 in, 2 out]
            n182 = property on="曲线模型" class="Clust (严格)"() -> ("Value"=w247:T2)  [unwired: 2 in, 2 out]
            n183 = case shown="\"标样核查\"" w248 {
              tunnel: w247 -> [_ w255 w257 w259 w261 w263]
              tunnel: [_ w254 w256 w258 w260 w262] -> w246
              frame "未选择", Default {
              }
              frame "空白校准" {
                n184 = Unbundle By Name(w255) -> ("标液浓度1"=w254:dbl)
              }
              frame "标样校准" {
                n185 = Unbundle By Name(w257) -> ("标液浓度2"=w256:dbl)
              }
              frame "标样核查" {
                n186 = Unbundle By Name(w259) -> ("标液浓度3"=w258:dbl)
              }
              frame "零点核查" {
                n187 = Unbundle By Name(w261) -> ("标液浓度4"=w260:dbl)
              }
              frame "跨度核查" {
                n188 = Unbundle By Name(w263) -> ("标液浓度5"=w262:dbl)
              }
            }
            n189 = Bundle By Name(cluster=w245, "id"=w250, "任务类型"=w248, "量程下拉列表"=w249, "标液浓度"=w246) -> (w244:T3)
            n190 = Generate User Event(user event=w251, event data cluster=w244) -> ()  [unwired: 2 in, 2 out]
          }
        }
      }
      event "历史数据导入": Value Change {
        n191 = event-data() -> ("NewVal"=w266:T1)  [unwired: 1 in, 5 out]
        n192 = Not Equal?(x=w266, y=T1."未选择") -> (x != y?=w267:bool)
        n193 = case shown="真" w267 {
          tunnel: w271 -> [_ _]
          tunnel: w270 -> [_ w281]
          tunnel: w269 -> [_ w274]
          tunnel: w266 -> [_ w272]
          tunnel: w265 -> [_ _]
          tunnel: w264 -> [_ w276]
          frame False {
          }
          frame True {
            n194 = property class="Enum (严格)"(reference=w274) -> ("Value"=w273:enum16{"低量程", "高量程"})  [unwired: 1 in, 2 out]
            n195 = property class="Ring (严格)"(reference=w281) -> ("Value"=w275:u16)  [unwired: 1 in, 2 out]
            n196 = property on="历史数据导入" class="RadioBtnsControl (严格)"("Value"=T1."未选择" ("历史数据导入")) -> ()  [unwired: 2 in, 2 out]
            n197 = call "id参数转换.vi"("id"=w275) -> ("table输出"=w280:string)  [unwired: 9 in, 1 out]
            n198 = call "校准数据选择表.vi"("测量模式"=w272, "量程下拉列表"=w273, "table"=w280) -> ("布尔"=w279:bool, "输出"=w278:T8)  [unwired: 7 in]
            n199 = case shown="真" w279 {
              tunnel: w278 -> [_ w289]
              tunnel: w272 -> [_ w291]
              tunnel: w276 -> [_ w290]
              tunnel: w275 -> [_ w288]
              tunnel: w273 -> [_ w287]
              frame False {
              }
              frame True {
                w285 = T3 {"id"=1, "任务类型"=enum."未选择", "量程下拉列表"=enum."低量程", "状态"=enum."已执行", "标液浓度"=0.0, "吸光值"=0.0, "校准时间"=timestamp(0 s since 1904-01-01)}  # 校准任务
                n200 = Unbundle By Name(w289) -> ("标液值"=w282:dbl, "吸光值"=w283:dbl, "时间"=w284:timestamp)
                n201 = Bundle By Name(cluster=w285, "id"=w288, "任务类型"=w291, "量程下拉列表"=w287, "标液浓度"=w282, "吸光值"=w283, "校准时间"=w284) -> (w286:T3)
                n202 = Generate User Event(user event=w290, event data cluster=w286) -> ()  [unwired: 2 in, 2 out]
              }
            }
          }
        }
      }
      event "校准任务": Value Change {
        n203 = event-data() -> ("NewVal"=w292:bool)  [unwired: 1 in, 5 out]
        n204 = invoke on="子面板" class="SubPnl" method="Remove VI"() -> (error out=w294:errorcluster)  [unwired: 3 in, 2 out]
        n205 = case shown="真" w292 {
          tunnel: w294 -> [_ w301]
          tunnel: w293 -> [_ w298]
          frame False {
          }
          frame True {
            n206 = vi-ref "校准任务设置.vi"() -> (w300:refnum<vi>)
            n207 = property class="VI"(reference=w300) -> (reference out=w296:refnum<vi>, "Name"=w299:string, "Exec.State"=w297:T9)  [unwired: 1 in, 1 out]
            n208 = case shown="\"Idle\"" w297 {
              tunnel: w299 -> [_ w313]
              tunnel: w298 -> [_ w310]
              tunnel: [w302 w306] -> w295
              tunnel: w296 -> [w302 w306]
              frame "Bad", Default {
              }
              frame "Idle" {
                n209 = Open VI Reference(type specifier VI Refnum (for type only)=refnum<vi> refnum, vi path=w313, options=128 ("选项")) -> (vi reference=w311:refnum<vi>, error out=w308:errorcluster)  [unwired: 3 in]
                n210 = property on="模型" class="Enum (严格)"() -> ("Value"=w304:enum32{"线性", "多项式"})  [unwired: 2 in, 2 out]
                n211 = property on="精度" class="DigNum (严格)"() -> ("Value"=w303:dbl)  [unwired: 2 in, 2 out]
                n212 = call-by-ref "开始异步调用"(reference=w311, error in=w308, "精度"=w303, "模型"=w304, "用户事件"=w310) -> (reference out=w309:refnum<vi>, error out=w307:errorcluster)  [unwired: 9 in]
                n213 = Close Reference(reference=w309, error in (no error)=w307) -> ()  [unwired: 1 out]
              }
            }
            n214 = invoke on="子面板" class="SubPnl" method="Insert VI"(error in=w301, "VI Ref"=w295) -> ()  [unwired: 2 in, 4 out]
          }
        }
      }
    }
  }
